vi "Filter.vi"(8 "error in":errorcluster, 9 "Image.Image original":T1, 10 "Image.Image copy":T1, 11 "Session Config":T2) -> (0 "error out":errorcluster, 1 "Session Out":T2, 2 "Data":string, 3 "Image Out":T1)   [LabVIEW 2020]
uses:
  <vilib>/userdefined/High Color/IMAQdx.ctl
  <vilib>/vision/Image Controls.llb/IMAQ Image.ctl
  <vilib>/vision/driver/IMAQdx.llb/IMAQdx Buffer Number Mode.ctl
  <vilib>/vision/NI_Vision_Development_Module.lvlib
  <vilib>/vision/driver/NI_Vision_Acquisition_Software.lvlib
panel:
  out "Image":T1(plugin-control)
  out "Found?":bool
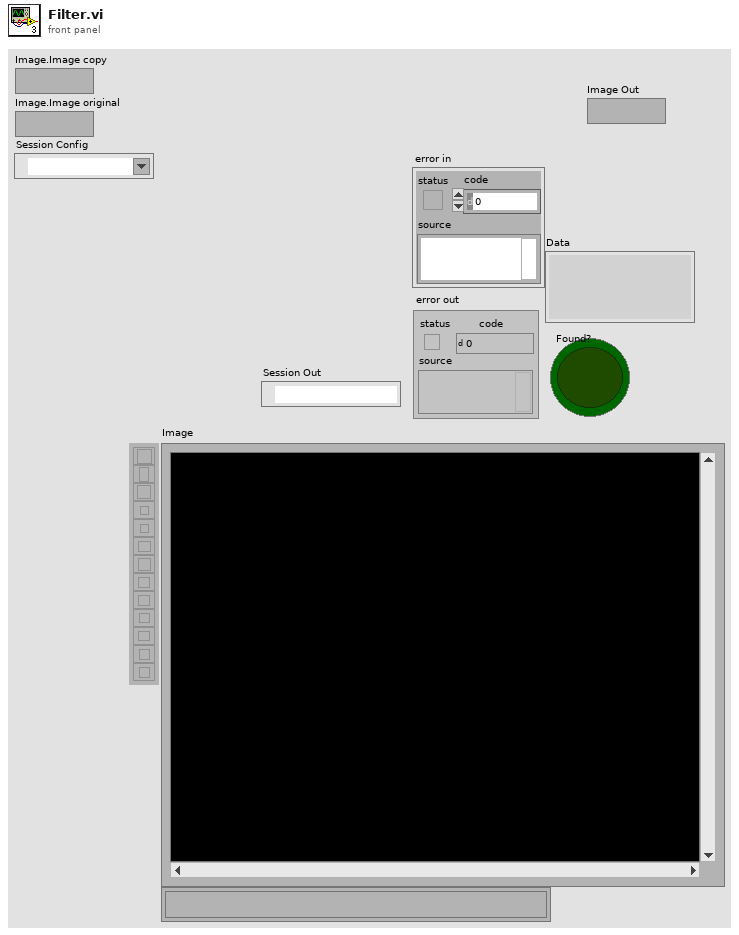
[diagram p1: front panel]
types:
  T1 = typedef "IMAQ Image.ctl" = refnum<image>
  T2 = typedef "IMAQdx.ctl" = refnum<k21>
  T3 = typedef "NI_Vision_Acquisition_Software.lvlib/IMAQdx Buffer Number Mode.ctl" = enum32{"Next", "Last", "Buffer Number", "Every", "Last New"}
  T4 = cluster{"Session Config":T2, "Image":cluster{"Image original":T1, "Image copy":T1}, "error in":errorcluster}
  T5 = typedef "QR Code Report.ctl" = cluster{"Found?":bool, "Data":string, "Bounding Box":cluster{"x":sgl, "y":sgl}[], "Errors Corrected":u32, "Dimensions (Rows/Cols)":u32, "Version":u32, "QR Model":T6, "Stream Mode":T7, "Barcode Polarity":T8, "Mirrored?":bool, "Append Stream Position":u32, "Size of Append Stream":u32, "First EAN-128 ID":i32, "First Alternate Language ID":i32, "Append Stream ID":u32, "Minimum Edge Strength":u32, "Demodulation Mode":T9, "Cell Sample Size":T10, "Cell Filter Mode":T11}
  T6 = typedef "QR Code Model Type.ctl" = i32
  T7 = typedef "QR Code Stream Mode Type.ctl" = i32
  T8 = typedef "Data Matrix Polarity.ctl" = i32
  T9 = typedef "Demodulation Mode.ctl" = i32
  T10 = typedef "Cell Sample Size.ctl" = i32
  T11 = typedef "Cell Filter Mode.ctl" = i32
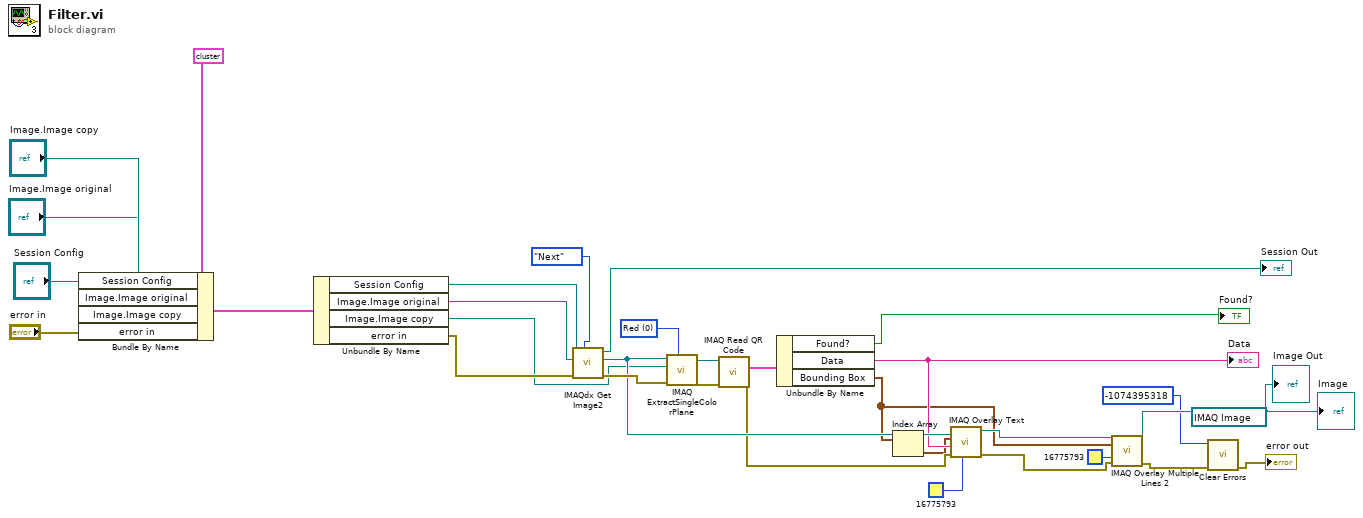
[diagram p0: block diagram]
diagram:
  (unwired) T1 refnum ("Image")
  w3 = 0 items=["Red", "Green", "Blue", "Hue", "Saturation", "Luminance", "Value", "Intensity"] ("Color Plane")
  n1 = Bundle By Name(cluster=T4 {"Session Config"="", "Image"={"Image original"=refnum, "Image copy"=refnum}, "error in"={"status"=FALSE, "code"=0, "source"=""}}, "Session Config"="Session Config", "Image.Image original"="Image.Image original", "Image.Image copy"="Image.Image copy", "error in"="error in") -> (w29:T4)
  n2 = Unbundle By Name(w29) -> ("Session Config"=w7:T2, "Image.Image original"=w8:T1, "Image.Image copy"=w2:T1, "error in"=w9:errorcluster)
  n3 = call <vilib>:"IMAQdx Get Image2.vi"("Buffer Number Mode (Next)"=IMAQdx_Buffer_Number_Mode."Next", "error in"=w9, "Image In"=w8, "Session In"=w7) -> ("error out"=w24:errorcluster, "Image Out"=w23:T1, "Session Out"=→"Session Out":T2)  [unwired: 4 in, 1 out]
  n4 = call "IMAQ ExtractSingleColorPlane"("Color Plane"=w3, "error in (no error)"=w24, "Image Dst"=w2, "Image Src"=w23) -> ("error out"=w11:errorcluster, "Image Dst Out"=w19:T1)  [unwired: 6 in]
  n5 = call "IMAQ Read QR Code"("error in (no error)"=w11, "Image"=w19) -> ("error out"=w17:errorcluster, "QR Code Report"=w12:T5)  [unwired: 6 in, 2 out]
  n6 = Unbundle By Name(w12) -> ("Found?"=→"Found?":bool, "Data"=w22:string, "Bounding Box"=w15:cluster{"x":sgl, "y":sgl}[])
  "Data" <- w22
  n7 = Index Array(array=w15) -> (element=w14:cluster{"x":sgl, "y":sgl})  [unwired: 1 in]
  n8 = call "IMAQ Overlay Text"("Text Color (black)"=u32 16775793, "error in (no error)"=w17, "String"=w22, "Origin"=w14, "Image"=w23) -> ("error out"=w16:errorcluster, "Image Out"=w18:T1)  [unwired: 5 in]
  n9 = call "IMAQ Overlay Multiple Lines 2"("Image"=w18, "Line End Points"=w15, "Color"=u32 16775793, "error in (no error)"=w16) -> ("Image Out"=→"Image" →"Image Out":T1, "error out"=w20:errorcluster)  [unwired: 10 in]
  n10 = call <vilib>:"Clear Errors.vi"("error in (no error)"=w20, "specific error code to clear (0: all)"=-1074395318) -> ("error out"=→"error out":errorcluster)  [unwired: 4 in, 1 out]
